vi "TestStand - GetLibraryName.vi"(10 "ProjectPath":string, 11 "BuildSpecification":string) -> (1 "error out":errorcluster, 2 "LibraryPath":string, 3 "LibraryName":string)   [LabVIEW 2023]
uses:
  <vilib>/AppBuilder/AB_API/common/AB_API Build Object Selector.ctl
  <vilib>/AppBuilder/AB_API/Build/NI_AB_API_Build.lvclass
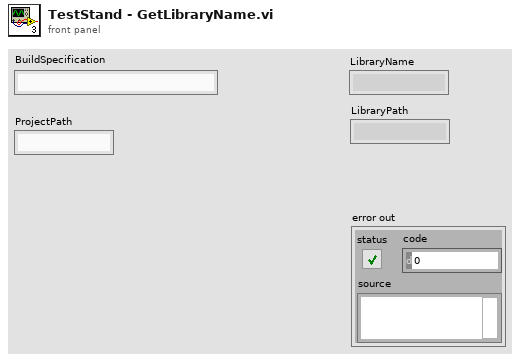
[diagram p1: front panel]
types:
  T1 = typedef "AB_API Build Object Selector.ctl" = enum16{"Source Distribution", "Deployable Source Distribution", "DLL", "EXE", "Packed Library", "Deployable Packed Library", "RT EXE", ".NET Interop Assembly"}
  T2 = typedef "AB_API Destination Data.ctl" = cluster{"Name":string, "Path":path, "Destination type":T3}
  T3 = typedef "AB_API Destination Type.ctl" = enum16{"directory", "directory (preserve hierarchy)", "LLB"}
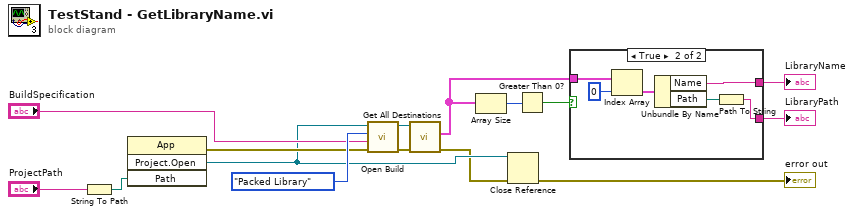
[diagram p0: block diagram]
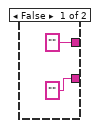
[diagram p2: hidden frame]
diagram:
  n1 = String To Path(string="ProjectPath") -> (path=w12:path)
  n2 = invoke class="App" method="Project.Open"("Path"=w12) -> (error out=w9:errorcluster, "Project:Open"=w8:refnum<vi>)  [unwired: 3 in, 2 out]
  n3 = call <vilib>:"Open Build.vi"("error in (no error)"=w9, "Build specification name"="BuildSpecification", "Build object selector"=AB_API_Build_Object_Selector."Packed Library", "Project Refnum"=w8) -> ("error out"=w10:errorcluster, "NI_AB_API_Build out"=w14:refnum<class "NI_AB_API_Build.lvclass">)  [unwired: 6 in]
  n4 = call-dynamic "Get All Destinations.vi"("error in (no error)"=w10, "NI_AB_API_Build in"=w14) -> ("error out"=w7:errorcluster, "Destinations"=w6:T2[])  [unwired: 7 in, 1 out]
  n5 = Array Size(array=w6) -> (size(s)=w2:i32)
  n6 = Close Reference(reference=w8, error in (no error)=w7) -> (error out=→"error out":errorcluster)
  n7 = Greater Than 0?(x=w2) -> (x > 0?=w1:bool)
  n8 = case shown="True" w1 {
    tunnel: w6 -> [_ w23]
    tunnel: ["" ("Name") w20] -> w5
    tunnel: ["" w18] -> w3
    frame False {
    }
    frame True {
      n9 = Index Array(array=w23, index=0) -> (element=w21:T2)
      n10 = Unbundle By Name(w21) -> ("Name"=w20:string, "Path"=w19:path)
      n11 = Path To String(path=w19) -> (string=w18:string)
    }
  }
  "LibraryName" <- w5
  "LibraryPath" <- w3
